vi "Vision Research Phantom Series PhCon PhSearchForAllCameras.vi"(5 "Error In (no error)":errorcluster, 9 "CallID":u32=1) -> (19 "Error Out":errorcluster)   [LabVIEW 2013, in "VRI.lvlib"]
doc: "PhCon.dll\n\nPhSearchForAllCameras\nHRESULT PhSearchForAllCameras(UINT CallID);\n\nParameters Description\nCallID (in) The call identifier (a number 1 to 15).\n Uses as a progress indicator parameter for calling\n PhLVProgress().\nReturn HRESULT (0 =Ok)\nComments Use this function to search for all cameras connected to\n the network of your computer regardless of the contents\n of the visible and ignored lists."
uses:
  VRI.lvlib
  Phantom DLLs/PhCon.Dll
panel:
  # "For instructions on the use of this VI, press Ctrl+H to display the help window and move the mouse over the icon, controls, and indicators"
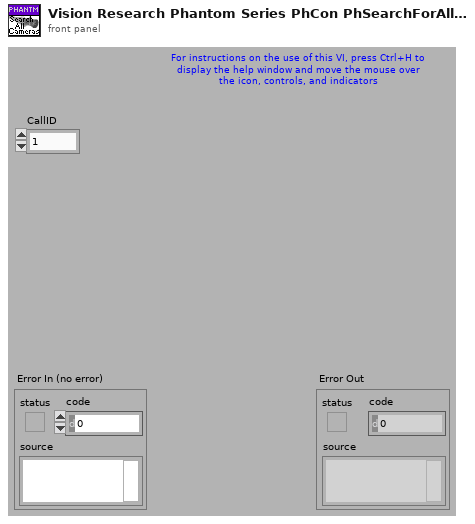
[diagram p1: front panel]
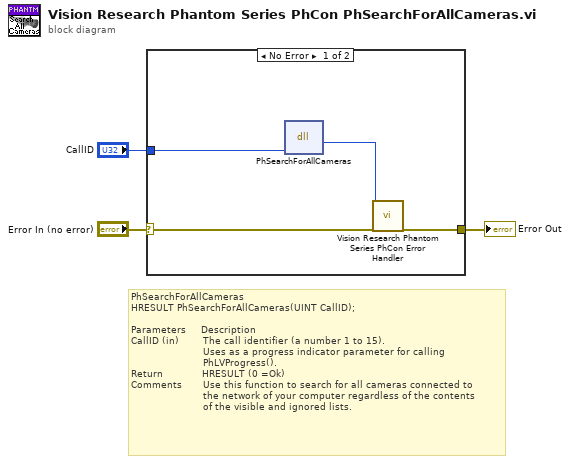
[diagram p0: block diagram]
diagram:
  # "PhSearchForAllCameras\nHRESULT PhSearchForAllCameras(UINT CallID);\n\nParameters     Description\nCallID (in)        The call identifier (a number 1 to 15).\n                        Uses as a progress indicator parameter for calling\n                        PhLVProgress().\nReturn             HRESULT (0 =Ok)\nComments       Use this function to search for all cameras connected to\n                        the network of your computer regardless of the contents\n                        of the visible and ignored lists."
  n1 = case shown="No Error" "Error In (no error)" {
    selector: "Error In (no error)" -> [w7 w8]
    tunnel: [w6 w8] -> w2
    tunnel: "CallID" -> [w5 _]
    frame No Error {
      n2 = dll-call lib="C:/Projects/SDK/64-bit/Vision Research Phantom Series Labview Driver/Phantom DLLs/PhCon.dll" fn="PhSearchForAllCameras"("CallID"=w5) -> ("HRESULT"=w4:i32)  [unwired: 4 in, 2 out]
      n3 = call "Vision Research Phantom Series PhCon Error Handler.vi"("ErrNo"=w4, "Error In (no error)"=w7) -> ("Error Out"=w6:errorcluster)  [unwired: 17 out]
    }
    frame Error {
    }
  }
  "Error Out" <- w2
